vi "Jog XY_o.vi"(10 "array IN":dbl[](array[numeric]), 11 "Jog Cluster":T1={"Jog XY Cluster"={"object goes up"=FALSE, "object goes down"=FALSE, "object goes right"=FALSE, "object goes left"=FALSE, "SW2"=FALSE, "SW1"=FALSE, "YY (mm)"=0.1, "YN (mm) "=0.01, "NY (mm) "=0.005, "NN (mm) "=0.001}, "Jog Z Cluster "={"Z go down 0.1 mm"=FALSE, "Z go up 0.1 mm"=FALSE, "Z go down 0.05 mm"=FALSE, "Z go up 0.05 mm"=FALSE, "Z go down 0.01 mm"=FALSE, "Z go up 0.01 mm"=FALSE, "Z go down"=FALSE, "Z go up"=FALSE, "step (mm)"=0.001}}) -> (2 "array OUT":dbl[](array[numeric]), 3 "Jog Cluster 2":T1={"Jog XY Cluster"={"object goes up"=FALSE, "object goes down"=FALSE, "object goes right"=FALSE, "object goes left"=FALSE, "SW2"=FALSE, "SW1"=FALSE, "YY (mm)"=0.1, "YN (mm) "=0.01, "NY (mm) "=0.005, "NN (mm) "=0.001}, "Jog Z Cluster "={"Z go down 0.1 mm"=FALSE, "Z go up 0.1 mm"=FALSE, "Z go down 0.05 mm"=FALSE, "Z go up 0.05 mm"=FALSE, "Z go down 0.01 mm"=FALSE, "Z go up 0.01 mm"=FALSE, "Z go down"=FALSE, "Z go up"=FALSE, "step (mm)"=0.001}})   [LabVIEW 2016]
panel:
  out "index of element":i32
  out "appended array":bool[](array[boolean])
  out "element":dbl
  out "floor(x/y)":dbl
  out "output array":dbl[](array[numeric])
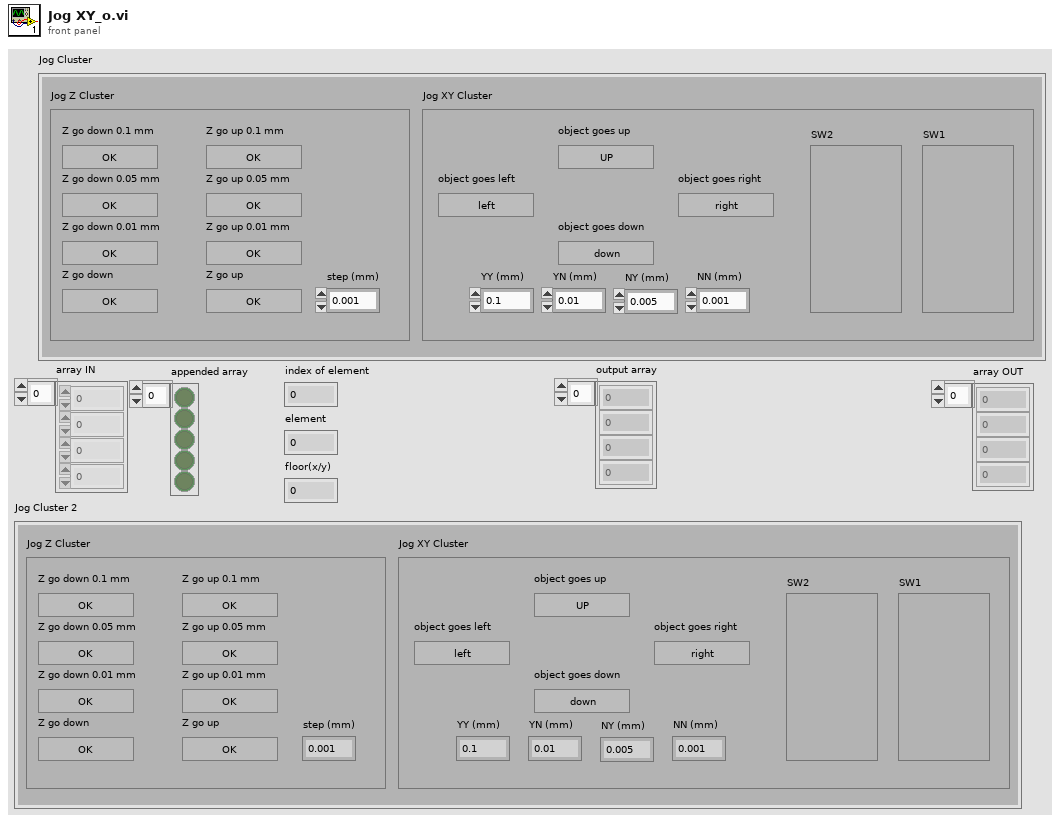
[diagram p1: front panel]
types:
  T1 = cluster{"Jog XY Cluster":cluster{"object goes up":bool, "object goes down":bool, "object goes right":bool, "object goes left":bool, "SW2":bool, "SW1":bool, "YY (mm)":dbl, "YN (mm) ":dbl, "NY (mm) ":dbl, "NN (mm) ":dbl}, "Jog Z Cluster ":cluster{"Z go down 0.1 mm":bool, "Z go up 0.1 mm":bool, "Z go down 0.05 mm":bool, "Z go up 0.05 mm":bool, "Z go down 0.01 mm":bool, "Z go up 0.01 mm":bool, "Z go down":bool, "Z go up":bool, "step (mm)":dbl}}
  T2 = cluster{"object goes up":bool, "object goes down":bool, "object goes right":bool, "object goes left":bool, "SW2":bool, "SW1":bool, "YY (mm)":dbl, "YN (mm) ":dbl, "NY (mm) ":dbl, "NN (mm) ":dbl}
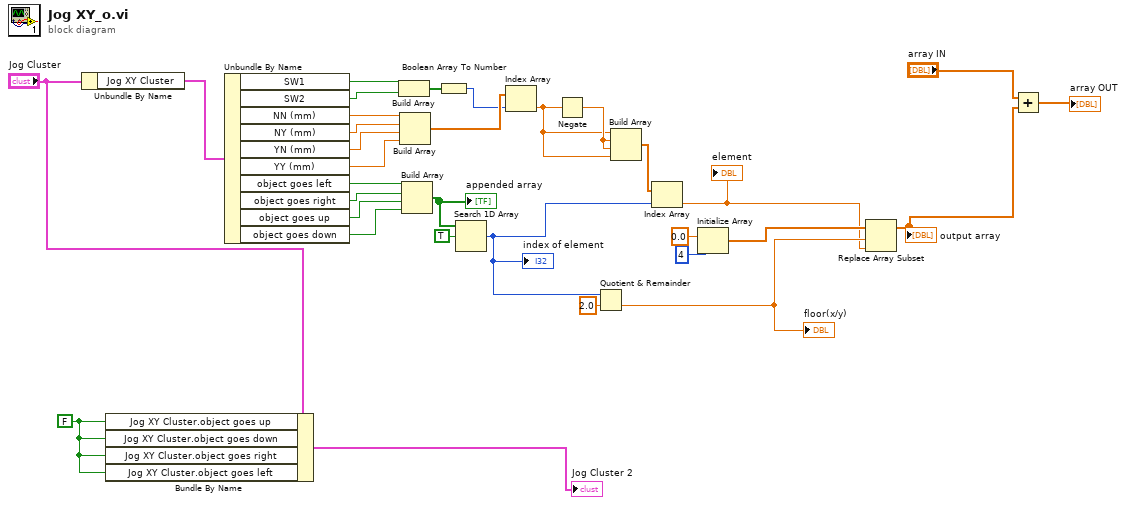
[diagram p0: block diagram]
diagram:
  w3 = FALSE ("Jog XY Cluster.object goes up")
  n1 = Unbundle By Name("Jog Cluster") -> ("Jog XY Cluster"=w30:T2)
  n2 = Bundle By Name(cluster="Jog Cluster", "Jog XY Cluster.object goes up"=w3, "Jog XY Cluster.object goes down"=w3, "Jog XY Cluster.object goes right"=w3, "Jog XY Cluster.object goes left"=w3) -> (→"Jog Cluster 2":T1)
  n3 = Unbundle By Name(w30) -> ("SW1"=w29:bool, "SW2"=w28:bool, "NN (mm)"=w27:dbl, "NY (mm)"=w26:dbl, "YN (mm)"=w25:dbl, "YY (mm)"=w24:dbl, "object goes left"=w20:bool, "object goes right"=w19:bool, "object goes up"=w18:bool, "object goes down"=w17:bool)
  n4 = Build Array(w29, w28) -> (w23:bool[])
  n5 = Build Array(w27, w26, w25, w24) -> (w22:dbl[])
  n6 = Build Array(w20, w19, w18, w17) -> (w8:bool[])
  "appended array" <- w8
  n7 = Boolean Array To Number(Boolean array=w23) -> (number=w21:u32)
  n8 = Search 1D Array(1D array=w8, element=TRUE) -> (index of element=w4:i32)  [unwired: 1 in]
  "index of element" <- w4
  n9 = Index Array(array=w22, index=w21) -> (element=w15:dbl)
  n10 = Negate(x=w15) -> (-x=w16:dbl)
  n11 = Quotient & Remainder(x=w4, y=2.0) -> (floor(x/y)=w10:dbl)  [unwired: 1 out]
  "floor(x/y)" <- w10
  n12 = Build Array(w15, w16, w16, w15) -> (w6:dbl[])
  n13 = Index Array(array=w6, index=w4) -> (element=w5:dbl)
  "element" <- w5
  n14 = Initialize Array(0.0 ("element"), 4 ("dimension size")) -> (w11:dbl[])
  n15 = Replace Array Subset(array=w11, new element=w5, index=w10) -> (w14:dbl[])
  "output array" <- w14
  n16 = Add(x="array IN", y=w14) -> (x+y=→"array OUT":dbl[])
